vi "Append Channel.vi"(8 "error in":errorcluster, 10 "Channel":string, 11 "BufferLastReads in":refnum<class "BufferLastReads.lvclass">) -> (0 "error out":errorcluster, 3 "BufferLastReads out":refnum<class "BufferLastReads.lvclass">)   [LabVIEW 2024, in "BufferLastReads.lvclass"]
uses:
  BufferLastReads.lvclass
  BufferLastReads.lvclass/BufferLastReads.ctl
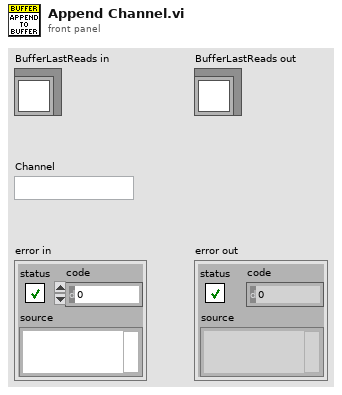
[diagram p1: front panel]
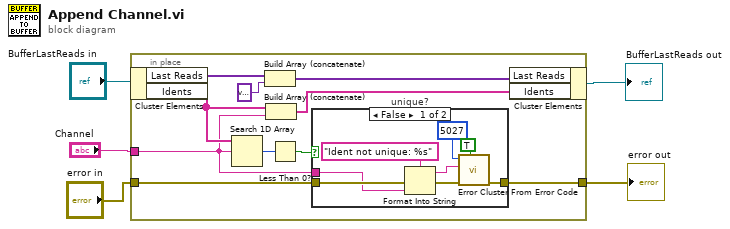
[diagram p0: block diagram]
diagram:
  n1 = in-place {
    in-place-border: [w13] -> w3
    in-place-border: "Channel" -> [w7]
    in-place-border: "error in" -> [w12]
    n2 = in-place-cluster #1("BufferLastReads in") -> ("Last Reads"=w11:variant[], "Idents"=w10:string[])
    n3 = Search 1D Array(1D array=w10, element=w7) -> (index of element=w14:i32)  [unwired: 1 in]
    n4 = Build Array (concatenate)(w11, variant) -> (w9:variant[])
    n5 = Build Array (concatenate)(w10, w7) -> (w8:string[])
    n6 = Less Than 0?(x=w14) -> (x < 0?=w15:bool)
    n7 = case "unique?" shown="False" w15 {
      tunnel: w12 -> [w23 w24]
      tunnel: [w22 w24] -> w13
      tunnel: w7 -> [w17 _]
      frame False {
        n8 = Format Into String(format string="Ident not unique: %s", error in=w23, w17) -> (resulting string=w16:string, error out=w19:errorcluster)  [unwired: 1 in]
        n9 = call <vilib>:"Error Cluster From Error Code.vi"("show call chain? (False)"=TRUE, "error in (no error)"=w19, "error message (\"\")"=w16, "error code (0)"=5027) -> ("error out"=w22:errorcluster)  [unwired: 5 in]
      }
      frame True {
      }
    }
    n10 = in-place-cluster #1("Last Reads"=w9, "Idents"=w8) -> (→"BufferLastReads out":refnum<class "BufferLastReads.lvclass">)
  }
  "error out" <- w3
